vi "WindToSailLookup.vi"(9 "DesiredProportionOfBoatSpeed":dbl, 10 "WindSpeed":dbl, 11 "ApparentWindAngle":dbl) -> (3 "Suggested Sail Setpoints":T1 {"MainSailSuggestion" min=0.0 max=1.0; "JibSailSuggestion" min=0.0 max=1.0})   [LabVIEW 2013]
doc: "Spring 2014\n\nInput: Relative Wind Angles\n\nReturns suggestions for the angle of the main sail and the angle of the jib sail, from a lookup table of relative wind to sail angles."
uses:
  Data/TypeDefs/Sail Set Suggestions.ctl
panel:
  # "TODO: Incorporate this data  later, see back\npanel for more information"
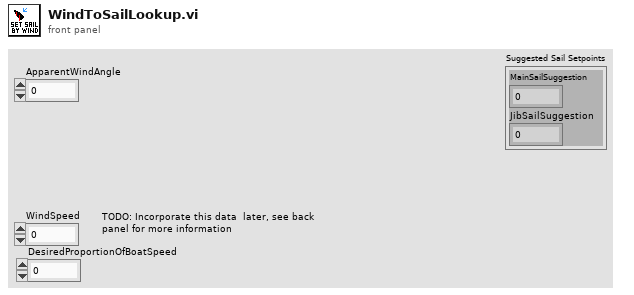
[diagram p1: front panel]
types:
  T1 = typedef "Sail Set Suggestions.ctl" = cluster{"MainSailSuggestion":dbl, "JibSailSuggestion":dbl}
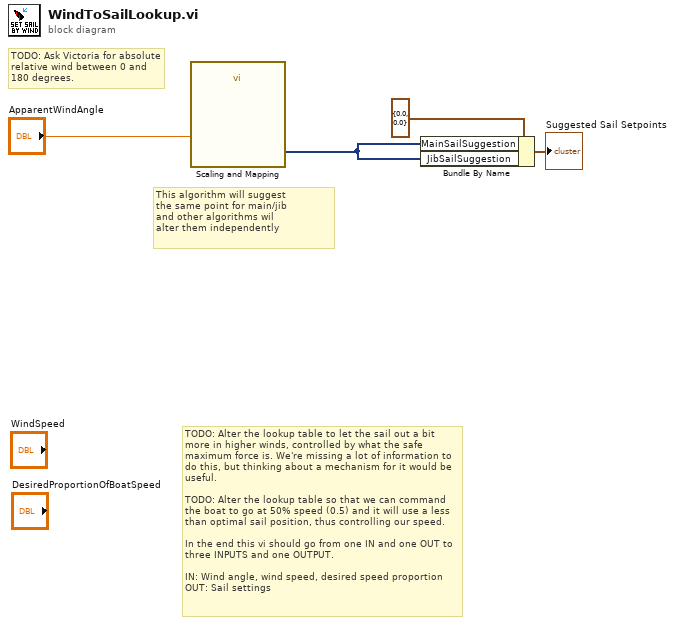
[diagram p0: block diagram]
diagram:
  # "TODO: Alter the lookup table to let the sail out a bit more in higher winds, controlled by what the safe maximum force is. We're missing a lot of information to do this, but thinking about a mechanism for it would be useful.\n\nTODO: Alter the lookup table so that we can command the boat to go at 50% speed (0.5) and it will use a less than optimal sail position, thus controlling our speed.\n\nIn the end this vi should go from one IN and one OUT to three INPUTS and one OUTPUT.\n\nIN: Wind angle, wind speed, desired speed proportion\nOUT: Sail settings"
  # "TODO: Ask Victoria for absolute\nrelative wind between 0 and\n180 degrees."
  # "This algorithm will suggest\nthe same point for main/jib\nand other algorithms wil\nalter them independently"
  n1 = call "Scaling and Mapping"("Signals"="ApparentWindAngle") -> ("Scaled Signals"=w1:dynamicdata)  [unwired: 9 in, 1 out]
  n2 = Bundle By Name(cluster=T1 {"MainSailSuggestion"=0.0, "JibSailSuggestion"=0.0} ("output cluster"), "MainSailSuggestion"=w1, "JibSailSuggestion"=w1) -> (→"Suggested Sail Setpoints":T1)
